vi "Timer.vi"(2 "Остановка процесса":bool, 8 "Рассчитанное время":dbl, 9 "shift before":u32) -> (0 "end time":bool, 1 "shift after":u32, 4 "Время с начала процесса":timestamp=timestamp(-10799.222 s since 1904-01-01) format="%<%H:%M:%S>T", 5 "Процесс выполнения (шкала)":dbl(slide) scale=0.0..1.0, 6 "Осталось времени \nдо конца процесса":timestamp=timestamp(-10799.186 s since 1904-01-01) format="%<%H:%M:%S>T")   [LabVIEW 2016]
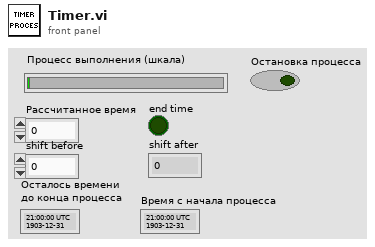
[diagram p1: front panel]
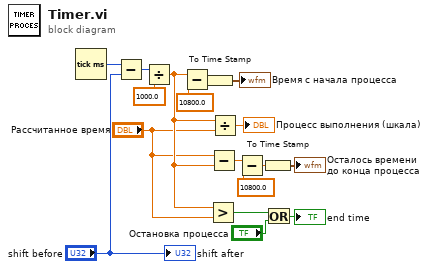
[diagram p0: block diagram]
diagram:
  n1 = Tick Count (ms)() -> (millisecond timer value=w17:u32)
  n2 = Subtract(x=w17, y="shift before") -> (x-y=w15:u32)
  n3 = Divide(x=w15, y=1000.0) -> (x/y=w6:dbl)
  n4 = Subtract(x=w6, y=10800.0) -> (x-y=w14:dbl)
  n5 = To Time Stamp(1:w14) -> (0:→"Время с начала процесса":timestamp)
  n6 = Greater?(x=w6, y="Рассчитанное время") -> (0:w3:bool)
  n7 = Subtract(x="Рассчитанное время", y=w6) -> (x-y=w8:dbl)
  n8 = Divide(x=w6, y="Рассчитанное время") -> (x/y=→"Процесс выполнения (шкала)":dbl)
  n9 = Subtract(x=w8, y=10800.0) -> (x-y=w7:dbl)
  n10 = To Time Stamp(1:w7) -> (0:→"Осталось времени \nдо конца процесса":timestamp)
  n11 = Or(x=w3, y="Остановка процесса") -> (x .or. y?=→"end time":bool)
  "shift after" <- "shift before"
